vi "PV Write-Read Core.vi"(4 "error in":errorcluster, 5 "Write data in":string, 7 "VISA session":refnum<visa-resource-name>) -> (0 "error out":errorcluster, 1 "response (data) out":string, 3 "dup VISA session":refnum<visa-resource-name>)   [LabVIEW 2024, in "Pfeiffer Vacuum.lvlib"]
uses:
  <instrlib>/Pfeiffer Vacuum/Pfeiffer Vacuum.lvlib
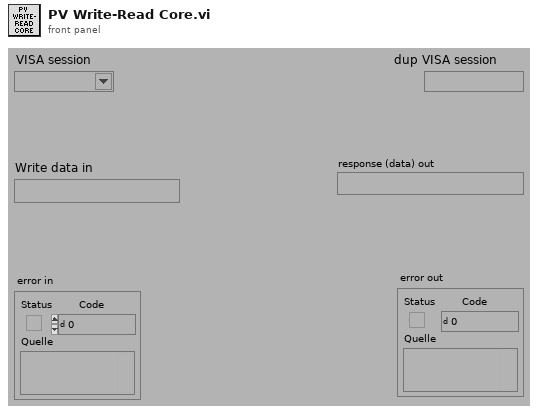
[diagram p1: front panel]
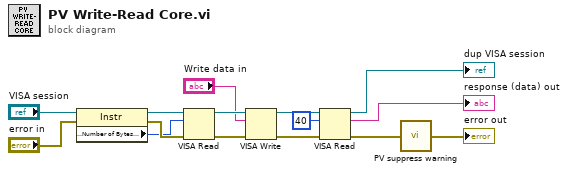
[diagram p0: block diagram]
diagram:
  n1 = property class="Instr"(reference="VISA session", error in="error in") -> (reference out=w12:refnum<visa-resource-name>, error out=w13:errorcluster, "Serial Settings:Number of Bytes at Serial Port"=w11:u32)
  n2 = VISA Read(VISA resource name=w12, byte count=w11, error in (no error)=w13) -> (VISA resource name out=w14:refnum<visa-resource-name>, error out=w6:errorcluster)  [unwired: 2 out]
  n3 = VISA Write(VISA resource name=w14, write buffer="Write data in", error in (no error)=w6) -> (VISA resource name out=w7:refnum<visa-resource-name>, error out=w5:errorcluster)  [unwired: 1 out]
  n4 = VISA Read(VISA resource name=w7, byte count=u32 40 ("Anzahl der Bytes (0)"), error in (no error)=w5) -> (VISA resource name out=→"dup VISA session":refnum<visa-resource-name>, read buffer=→"response (data) out":string, error out=w2:errorcluster)  [unwired: 1 out]
  n5 = call <instrlib>:"PV suppress warning.vi"("error in"=w2) -> ("error out"=→"error out":errorcluster)
